vi "4-1 Mux.vi"(0 "input 0":bool, 2 "select":u8, 5 "input 1":bool, 7 "input 2":bool, 9 "input 3":bool) -> (8 "output":bool)   [LabVIEW 2017]
doc: "Selects one of the 4 inputs based on the value of the select parameter."
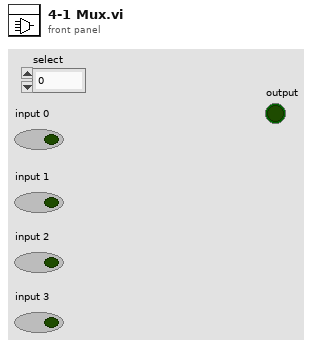
[diagram p1: front panel]
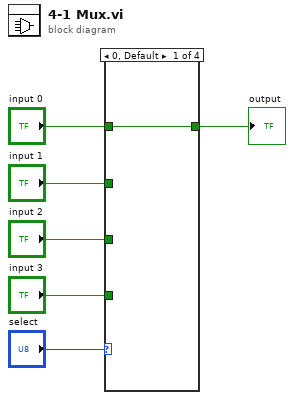
[diagram p0: block diagram]
diagram:
  n1 = case shown="0, Default" "select" {
    tunnel: "input 0" -> [w7 _ _ _]
    tunnel: "input 1" -> [_ w8 _ _]
    tunnel: "input 2" -> [_ _ w9 _]
    tunnel: "input 3" -> [_ _ _ w10]
    tunnel: [w7 w8 w9 w10] -> w2
    frame 0, Default {
    }
    frame 1 {
    }
    frame 2 {
    }
    frame 3 {
    }
  }
  "output" <- w2
